vi "Watt Noise Level.vi"() -> ()   [LabVIEW 2009]
uses:
  ChannelSettings.ctl
  <vilib>/Analysis/NI_AALBase.lvlib
panel:
  out "Time(mS),Watts":dbl[](array[numeric])
  out "standard deviation":dbl format="%0.2f"
  out "mean":dbl format="%0.2f"
  out "Histogram Graph":T1(graph)
  in  "Number of Samples":i32
  out "Watts":dbl(graph)
  out "error out":errorcluster
  out "Watts":dbl
  in  "milliseconds to wait":u32
  in  "error in (no error)":errorcluster
  in  "Semiphore":T2
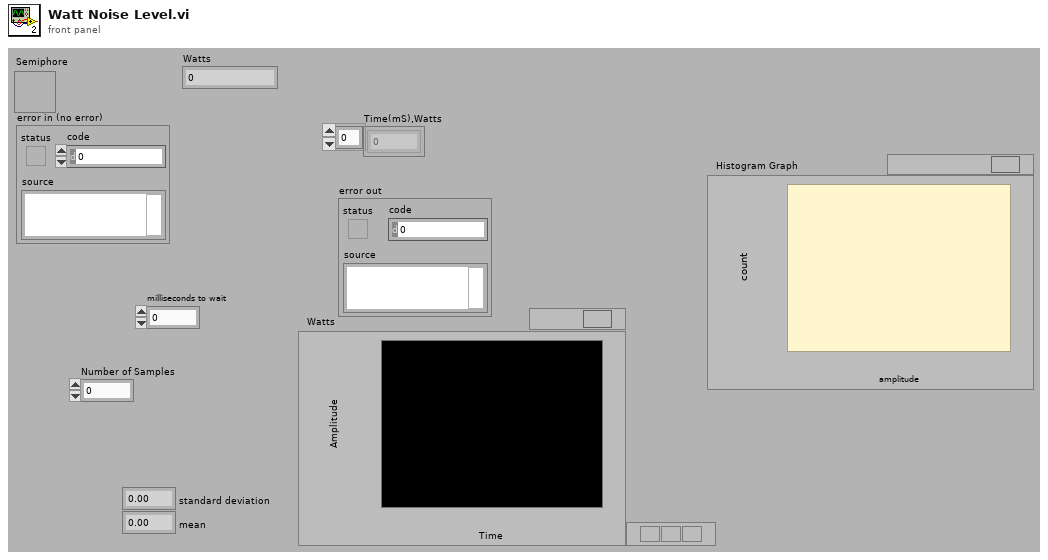
[diagram p1: front panel]
types:
  T1 = cluster{"X Values":dbl[], "Histogram: h(x)":i32[]}
  T2 = typedef "Semaphore RefNum" = refnum<k1>
  T3 = typedef "ChannelSettings.ctl" = u32
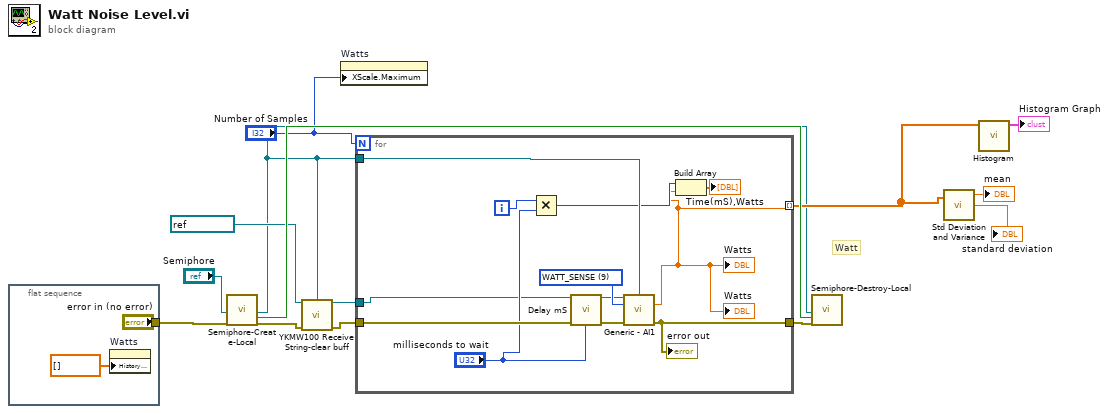
[diagram p0: block diagram]
diagram:
  # "Watt"
  n1 = flat-sequence {
    tunnel: ["error in (no error)"] -> w13
    frame #0 {
      n2 = property on="Watts" class="WFChart (strict)"("History Data"=dbl[] []) -> ()  [unwired: 2 in, 2 out]
    }
  }
  n3 = call "Semiphore-Create-Local.vi"("Semiphore"="Semiphore", "error in (no error)"=w13) -> ("semaphore"=w2:T2, "Local?"=w11:bool, "error out"=w5:errorcluster)  [unwired: 15 in]
  n4 = call "YKMW100 Receive String-clear buff.vi"("VISA session"=refnum<visa-resource-name> "MW100" ("MW100"), "Semiphore"=w2, "error in (no error)"=w5) -> ("dup VISA session"=w4:refnum<visa-resource-name>, "error out"=w6:errorcluster)  [unwired: 10 in, 1 out]
  n5 = property on="Watts" class="WFChart (strict)"("XScale.Maximum"="Number of Samples") -> ()  [unwired: 2 in, 2 out]
  n6 = for {
    N: "Number of Samples" -> [_]
    tunnel: w6 -> [w23]
    tunnel: w2 -> [w24]
    tunnel: [w25] -> w12
    tunnel: [w19] -> w9 mode=indexing
    tunnel: w4 -> [w17]
    i -> [w22]
    w27 = T3 9 items=["4-20_OUT", "Pres_HI1", "Pres_HI2", "Pres_LOW", "Pres_PIN", "HEATER_TOP", "HEATER_BOT", "T_Shell", "FLOWMETER", "WATT_SENSE", "WH_TICK", "Tc_1", "Tc_2", "Tc_3", "Tc_4", "Tc_5", "Tc_6", "Tc_down", "T_Shell_2", "T_Shell_3", "T_Shell_4", "RTD_IN", "RTD_OUT", "RTD_AMB", "INTF_TEMPFLO", "INTF_READY", "INTF_START", "INTF_STOP", "DRM_LOW", "DRM_HIGH", "PWR_MAIN", "VLV_DUMP", "VLV_OUT", "VLV_IN", "WATT_HOURS", "FLOW(SAMPLE)", "GALLONS", "FLOW(GPM)"] ("Channel_Enum")
    n7 = Multiply(x=w22, y="milliseconds to wait") -> (x*y=w20:u32)
    n8 = call "Delay mS.vi"("Error In"=w23, "milliseconds to wait"="milliseconds to wait") -> ("Error Out"=w26:errorcluster)  [unwired: 13 in]
    n9 = call "Generic - AI1.vi"("MW100"=w17, "Semiphore"=w24, "Channel_Enum"=w27, "Error In"=w26) -> ("Value"=w19:dbl, "Error Out"=w25:errorcluster)  [unwired: 9 in, 1 out]
    "Watts" <- w19
    "error out" <- w25
    "Watts" <- w19
    n10 = Build Array(w20, w19) -> (→"Time(mS),Watts":dbl[])
  }
  n11 = call "Semiphore-Destroy-Local.vi"("Semiphore"=w2, "Local?"=w11, "error in (no error)"=w12) -> ()  [unwired: 16 in, 1 out]
  n12 = call <vilib>:"Std Deviation and Variance.vi"("X"=w9) -> ("mean"=→"mean":dbl, "standard deviation"=→"standard deviation":dbl)  [unwired: 1 in, 1 out]
  n13 = call <vilib>:"Histogram.vi"("X"=w9) -> ("Histogram Graph"=→"Histogram Graph":T1)  [unwired: 7 in, 3 out]
